vi "ConstrainOutput.vi"(10 "Position [deg]":dbl, 11 "Motor Current Setpoint [V]":dbl) -> (3 "Motor Output":dbl)   [LabVIEW 2019]
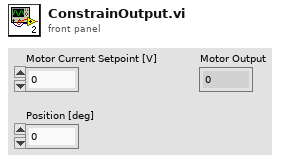
[diagram p1: front panel]
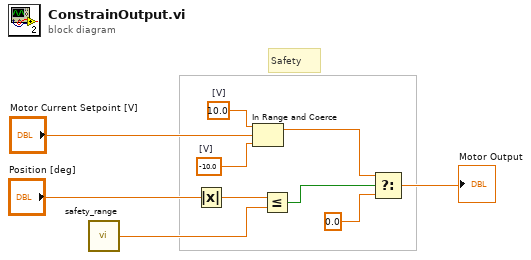
[diagram p0: block diagram]
diagram:
  w3 = -10.0  # [V]
  w4 = 10.0  # [V]
  # "Safety"
  n1 = call "safety_range.vi"() -> ("Safety Range"=w1:dbl)  [unwired: 2 in]
  n2 = Absolute Value(x="Position [deg]") -> (abs(x)=w6:dbl)
  n3 = In Range and Coerce(upper limit=w4, x="Motor Current Setpoint [V]", lower limit=w3) -> (coerced(x)=w5:dbl)  [unwired: 1 out]
  n4 = Less Or Equal?(x=w6, y=w1) -> (x <= y?=w7:bool)
  n5 = Select(t=w5, s=w7, f=0.0) -> (s? t:f=→"Motor Output":dbl)
